vi "Spatial Event Example.vi"() -> ()   [LabVIEW 2012, in "Phidget Spatial.lvlib"]
uses:
  <instrlib>/Phidgets/Phidget Spatial/Phidget Spatial.lvlib
  <instrlib>/Phidgets/Phidget Spatial/Public/SpatialStart.vi
  <instrlib>/Phidgets/Phidget Spatial/Public/SpatialClose.vi
  <instrlib>/Phidgets/Phidget Common/Phidget Common.lvlib
panel:
  out "Timestamp":u64
  out "Mag Field Data":dbl[](array[numeric]) caption="Field Str Data"
  out "Gyro Data":dbl[](array[numeric])
  out "Accel Data":dbl[](array[numeric])
  in  "stop":bool
  out "Serial Number Return":i32
  in  "Device Info":T1={"Serial Number"=-1, "Channel"=0, "Port"=0}
  out "error out":errorcluster
  # "Be sure to use this stop button to stop the program.\nIf you use the \"Abort Execution\" button, you will\nneed to use PhidgetResetLibrary.vi or restart Labview \nin order for any Phidgets to work."
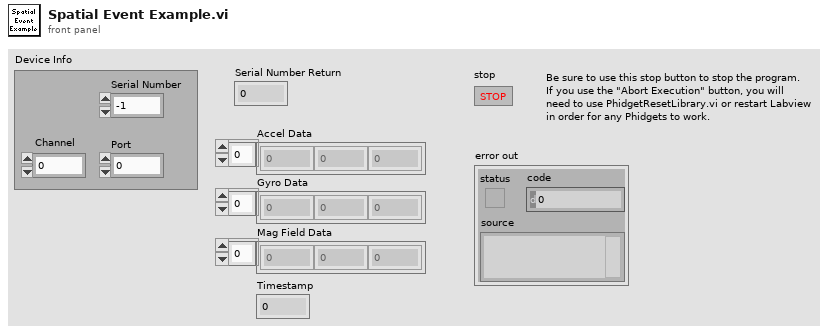
[diagram p1: front panel]
types:
  T1 = cluster{"Serial Number":i32, "Channel":i32, "Port":i32}
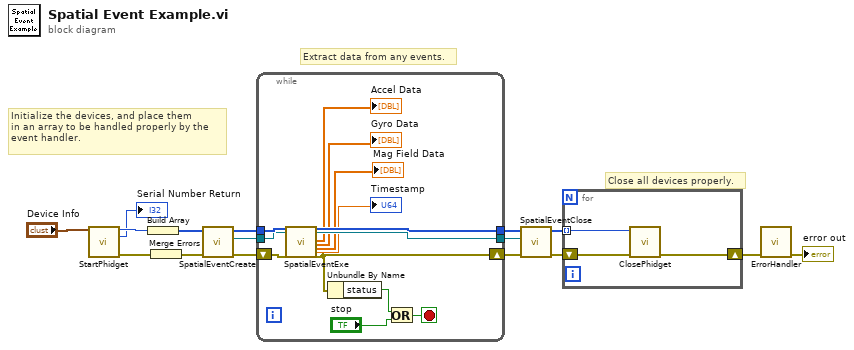
[diagram p0: block diagram]
diagram:
  # "Close all devices properly."
  # "Extract data from any events."
  # "Initialize the devices, and place them\nin an array to be handled properly by the\nevent handler."
  n1 = call-poly <instrlib>:"StartPhidget.vi"("Device Info"="Device Info") -> ("Phidget ID"=w5:u64, "Serial Number Return"=→"Serial Number Return":i32, "error out"=w2:errorcluster)  [unwired: 11 in, 1 out]
  n2 = Build Array(w5) -> (w16:u64[])
  n3 = Merge Errors(w2) -> (w7:errorcluster)
  n4 = call <instrlib>:"SpatialEventCreate.vi"("error in (no error)"=w7, "Devices In"=w16) -> ("error out"=w9:errorcluster, "Event Registration Refnum"=w14:refnum<event-registration>, "Devices Out"=w15:u64[])  [unwired: 7 in]
  n5 = while {
    tunnel: w15 -> [w29]
    tunnel: w14 -> [w25]
    tunnel: [w28] -> w11
    shift-right: [w24] -> w10
    shift-left: w9 -> [w27]
    tunnel: [w26] -> w3
    stop <- w23 stop-if-true
    n6 = call <instrlib>:"SpatialEventExe.vi"("Devices In"=w29, "Event Registration Refnum In"=w25, "error in (no error)"=w27) -> ("Devices Out"=w26:u64[], "Event Registration Refnum Out"=w28:refnum<event-registration>, "Accel Data"=→"Accel Data":dbl[], "Gyro Data"=→"Gyro Data":dbl[], "Field Str Data"=→"Mag Field Data":dbl[], "Timestamp"=→"Timestamp":dbl, "error out"=w24:errorcluster)  [unwired: 15 in, 3 out]
    n7 = Unbundle By Name(w24) -> ("status"=w21:bool)
    n8 = Or(x=w21, y="stop") -> (x .or. y?=w23:bool)
  }
  n9 = call <instrlib>:"SpatialEventClose.vi"("error in (no error)"=w10, "Event Registration Refnum In"=w11, "Devices In"=w3) -> ("error out"=w6:errorcluster, "Devices Out"=w4:u64[])  [unwired: 7 in]
  n10 = for {
    tunnel: w4 -> [w30] mode=indexing
    shift-right: [w32] -> w13
    shift-left: w6 -> [w31]
    n11 = call-poly <instrlib>:"ClosePhidget.vi"("error in"=w31, "Device In"=w30) -> ("error out"=w32:errorcluster)  [unwired: 9 in]
  }
  n12 = call <instrlib>:"ErrorHandler.vi"("error in"=w13) -> ("error out"=→"error out":errorcluster)  [unwired: 9 in, 1 out]
